vi "ABR-Options Dialog.vi"(0 "Params in":T3={"CAP or ABR"=enum."CAP", "Stimulus"={"Destination"="", "Waveform"=enum."TONE PIP", "Frequency (kHz)"=16.0, "Rep rate (/sec)"=30.0, "Alternate Polarity"=FALSE, "Sampling rate (Hz)"=0.0, "Duration (ms)"=30.0, "Ramp (ms)"=5.0, "Click width (us)"=0.0, "ITI"=enum."Rate", "Save raw"=FALSE}, "Sequence"={"Start (dB)"=20, "Stop (dB)"=80, "Step (dB)"=5}, "Response"={"Gain"=10000, "Averages"=512, "Window (ms)"=8.5, "Thr Fast Steps"=8.5, "Sampling rate (Hz)"=25000.0}} {"Sequence"."Start (dB)" step=5; "Response"."Thr Fast Steps" format="%.2f"; "Response"."Window (ms)" format="%.2f"; "Stimulus"."Frequency (kHz)" format="%.2f"}, 2 "Parent VI":refnum<vi>, 5 "Threshold Estimation In":T2) -> (4 "Params out":T3={"CAP or ABR"=enum."CAP", "Stimulus"={"Destination"="", "Waveform"=enum."TONE PIP", "Frequency (kHz)"=16.0, "Rep rate (/sec)"=30.0, "Alternate Polarity"=FALSE, "Sampling rate (Hz)"=0.0, "Duration (ms)"=30.0, "Ramp (ms)"=5.0, "Click width (us)"=0.0, "ITI"=enum."Rate", "Save raw"=FALSE}, "Sequence"={"Start (dB)"=20, "Stop (dB)"=80, "Step (dB)"=5}, "Response"={"Gain"=10000, "Averages"=512, "Window (ms)"=8.5, "Thr Fast Steps"=8.5, "Sampling rate (Hz)"=25000.0}} {"Sequence"."Start (dB)" step=5; "Response"."Thr Fast Steps" format="%.2f"; "Response"."Window (ms)" format="%.2f"; "Stimulus"."Frequency (kHz)" format="%.2f"}, 6 "Threshold Estimation Out":T2, 8 "Canceled?":bool)   [LabVIEW 2020]
uses:
  Typedefs/ABR-Parameters.ctl
  Typedefs/ABR-Stimulus.ctl
  Typedefs/ABR-Sequence.ctl
  Typedefs/ABR-Response.ctl
  Threshold Estimation VIs/ABR3-Threshold Estimation Parameters.ctl
  epl-vi-lib/Utility VIs/Buttons/KCheckmarkBoolean 2.ctl
panel:
  in  "Save raw data":T1
  out "exit signal":bool
  in  "ITI":enum16{"Rate", "Interval"}(ring) caption="Express intertrial timing as"
  in  "AI Fs":dbl caption="Input sampling rate (Hz)"
  in  "R2 criterion":dbl caption="Adj R2 criterion"
  in  "CC criterion":dbl caption="Corrcoef criterion"
  in  "Thr Tmax":dbl caption="Tmax (ms)"
  in  "Thr Tmin":dbl caption="Tmin (ms)"
  in  "ClickWidth":dbl caption="Click duration (us)"
  in  "ToneRamp":dbl caption="Tone burst ramp length (ms)"
  in  "ToneDur":dbl caption="Tone burst duration (ms)"
  in  "AO Fs":dbl caption="Output sampling rate (Hz)"
  in  "Cancel":bool
  in  "OK":bool
  # "Threshold estimation"
  # "Warning! Unless you're sure you know what you're doing, don't change these parameters"
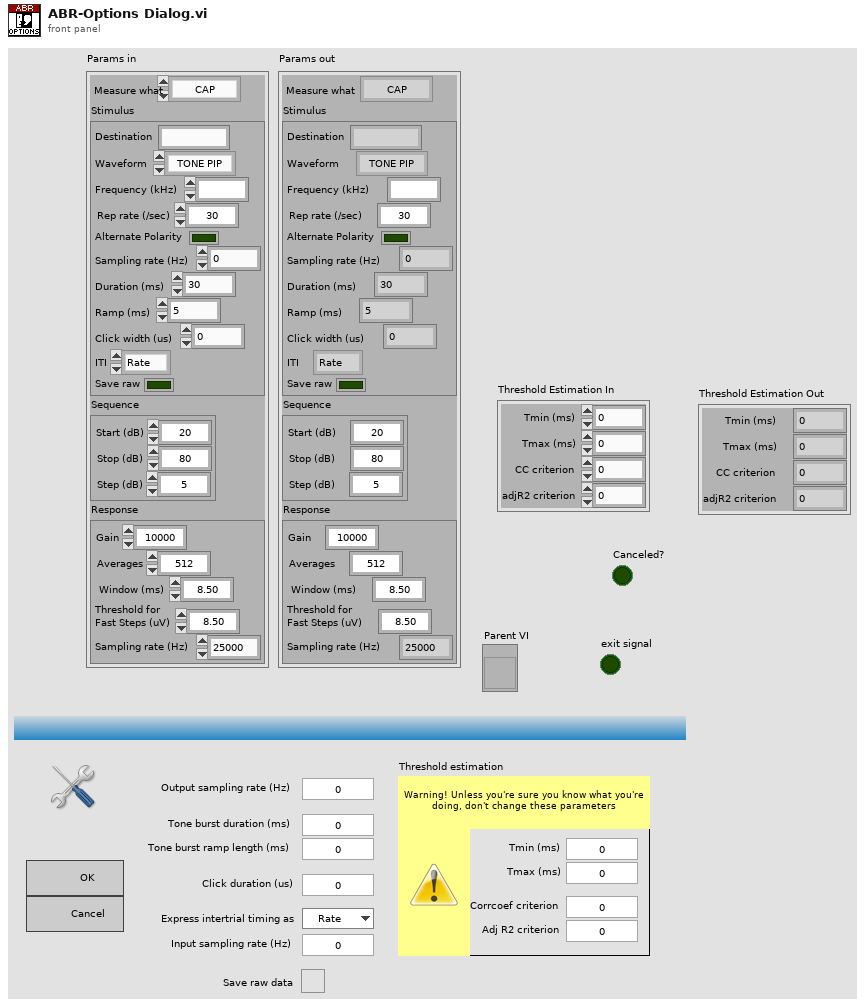
[diagram p1: front panel]
types:
  T1 = typedef "KCheckmarkBoolean 2.ctl" = bool
  T2 = typedef "ABR3-Threshold Estimation Parameters.ctl" = cluster{"Tmin (ms)":dbl, "Tmax (ms)":dbl, "CC criterion":dbl, "adjR2 criterion":dbl}
  T3 = typedef "ABR-Parameters.ctl" = cluster{"CAP or ABR":enum16{"CAP", "ABR"}, "Stimulus":T4, "Sequence":T5, "Response":T6}
  T4 = typedef "ABR-Stimulus.ctl" = cluster{"Destination":string, "Waveform":enum16{"TONE PIP", "CLICK"}, "Frequency (kHz)":ext, "Rep rate (/sec)":dbl, "Alternate Polarity":bool, "Sampling rate (Hz)":dbl, "Duration (ms)":dbl, "Ramp (ms)":dbl, "Click width (us)":dbl, "ITI":enum16{"Rate", "Interval"}, "Save raw":bool}
  T5 = typedef "ABR-Sequence.ctl" = cluster{"Start (dB)":i32, "Stop (dB)":i32, "Step (dB)":i32}
  T6 = typedef "ABR-Response.ctl" = cluster{"Gain":i32, "Averages":i32, "Window (ms)":sgl, "Thr Fast Steps":sgl, "Sampling rate (Hz)":dbl}
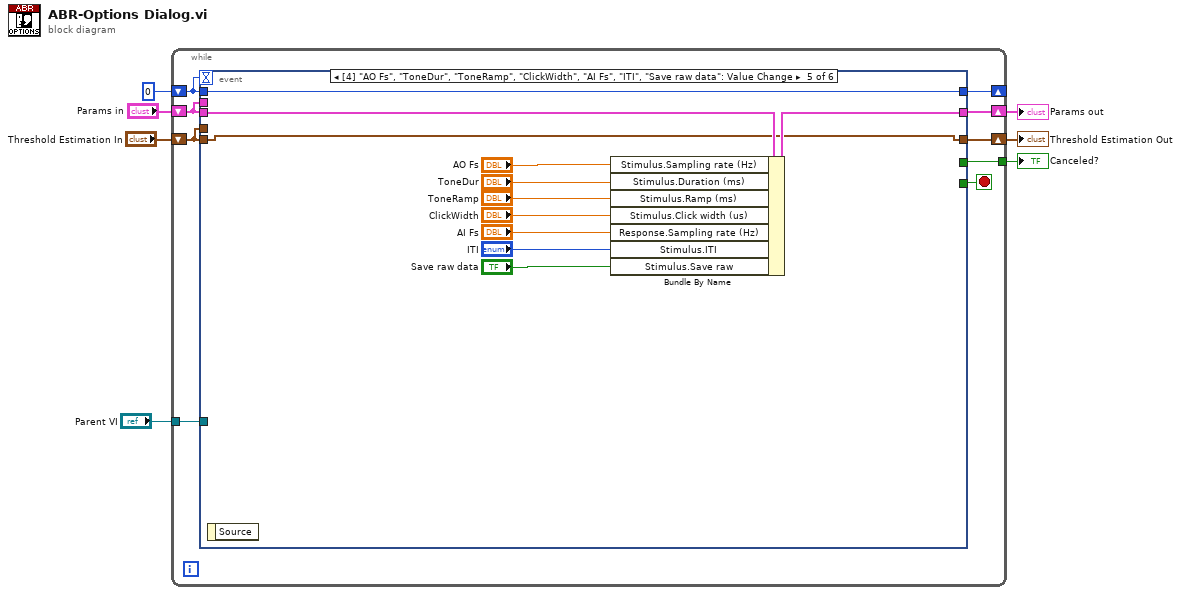
[diagram p0: block diagram]
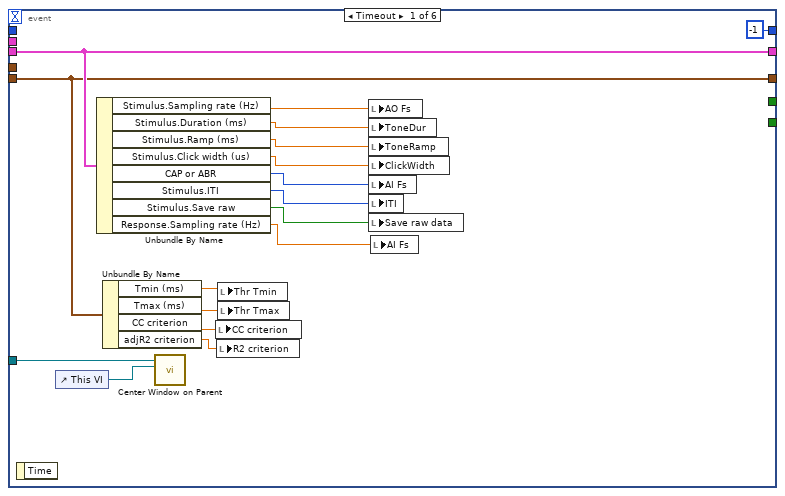
[diagram p2: hidden frame]
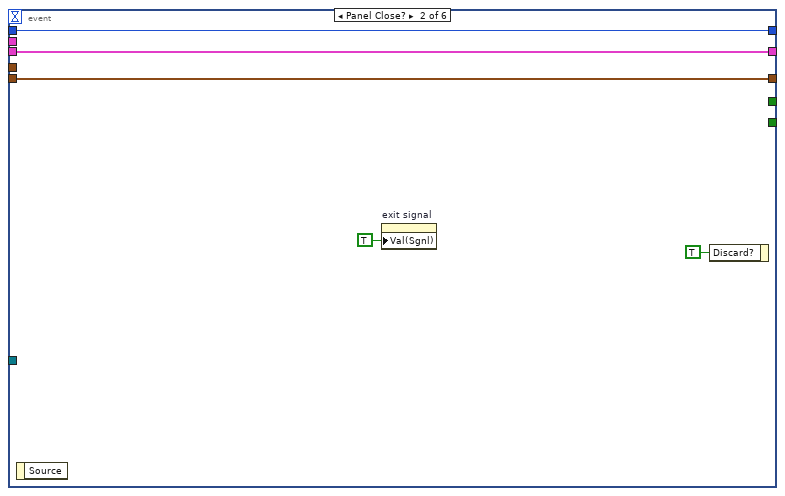
[diagram p3: hidden frame]
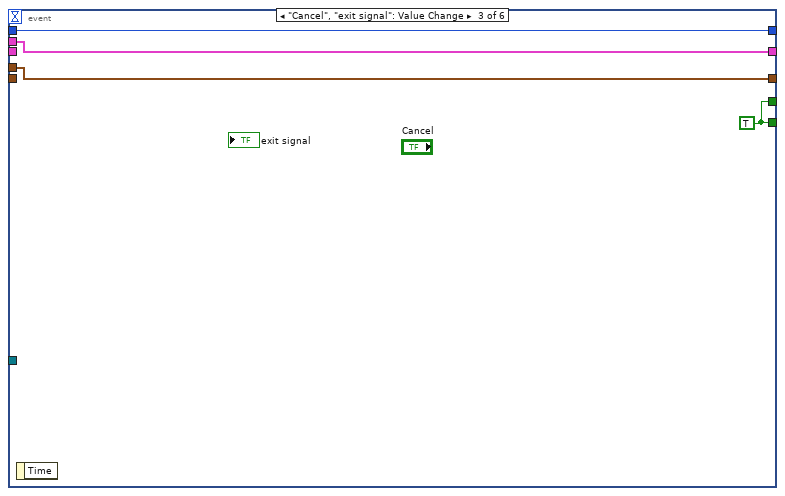
[diagram p4: hidden frame]
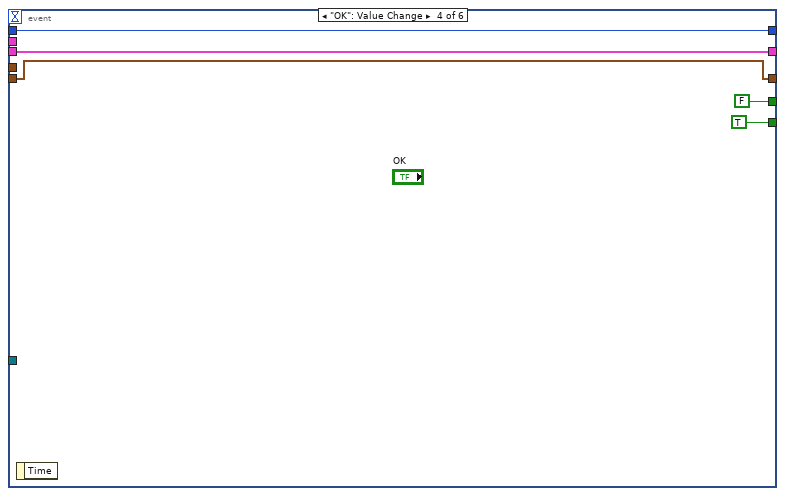
[diagram p5: hidden frame]
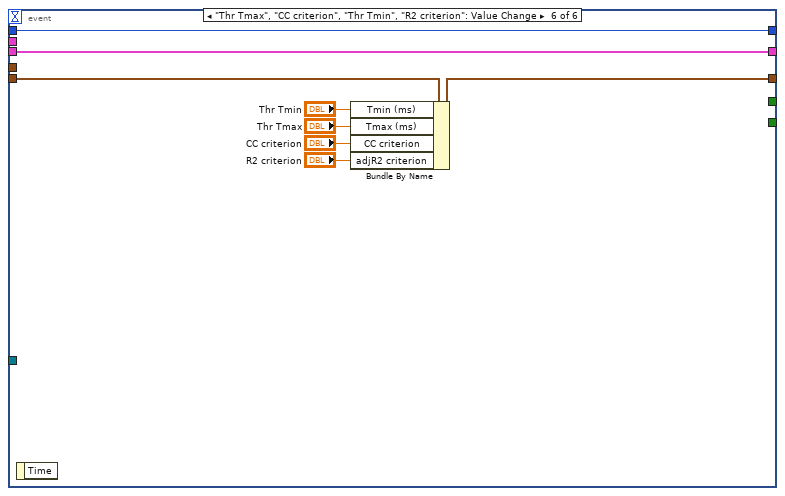
[diagram p6: hidden frame]
diagram:
  n1 = while {
    shift-right: [w16] -> _
    shift-left: 0 -> [w9]
    tunnel: [w13] -> w4
    shift-right: [w15] -> w5
    shift-left: "Params in" -> [w12]
    shift-right: [w11] -> w2
    shift-left: "Threshold Estimation In" -> [w10]
    tunnel: "Parent VI" -> [w8]
    stop <- w14 stop-if-true
    n2 = event shown="[4] \"AO Fs\", \"ToneDur\", \"ToneRamp\", \"ClickWidth\", \"AI Fs\", \"ITI\", \"Save raw data\": Value Change" {
      selector: _ -> [_ _ _ _ _ _]
      dyn-events: _ -> [_ _ _ _ _ _]
      timeout: w9 -> [_ _ _ _ _ _]
      tunnel: [-1 w38 w39 w43 w51 w62] -> w16
      tunnel: w12 -> [w32 w34 _ w47 w58 w66]
      tunnel: [w32 w34 w41 w47 w57 w66] -> w15
      tunnel: [_ _ w42 TRUE _ _] -> w14
      tunnel: [_ _ w42 FALSE _ _] -> w13
      tunnel: w12 -> [_ _ w41 _ _ _]
      tunnel: w10 -> [w27 w37 _ w44 w52 w60]
      tunnel: [w27 w37 w40 w44 w52 w59] -> w11
      tunnel: w10 -> [_ _ w40 _ _ _]
      tunnel: w9 -> [_ w38 w39 w43 w51 w62]
      tunnel: w8 -> [w23 _ _ _ _ _]
      event Timeout {
        n3 = event-data() -> ()  [unwired: 1 in, 1 out]
        n4 = control-ref of="This VI"() -> (w22:refnum<vi>)
        n5 = Unbundle By Name(w32) -> ("Stimulus.Sampling rate (Hz)"=w31:dbl, "Stimulus.Duration (ms)"=w30:dbl, "Stimulus.Ramp (ms)"=w29:dbl, "Stimulus.Click width (us)"=w28:dbl, "CAP or ABR"=w20:enum16{"CAP", "ABR"}, "Stimulus.ITI"=w19:enum16{"Rate", "Interval"}, "Stimulus.Save raw"=w18:bool, "Response.Sampling rate (Hz)"=w17:dbl)
        n6 = Unbundle By Name(w27) -> ("Tmin (ms)"=w26:dbl, "Tmax (ms)"=w25:dbl, "CC criterion"=w24:dbl, "adjR2 criterion"=w21:dbl)
        n7 = call "Center Window on Parent.vi"("Parent VI"=w22, "VI in"=w23) -> ()  [unwired: 8 in, 2 out]
        n8 = local write "CC criterion"(w24) -> ()
        n9 = local write "R2 criterion"(w21) -> ()
        n10 = local write "Thr Tmin"(w26) -> ()
        n11 = local write "Thr Tmax"(w25) -> ()
        n12 = local write "AO Fs"(w31) -> ()
        n13 = local write "ToneDur"(w30) -> ()
        n14 = local write "ToneRamp"(w29) -> ()
        n15 = local write "ClickWidth"(w28) -> ()
        n16 = local write "AI Fs"(w20) -> ()
        n17 = local write "ITI"(w19) -> ()
        n18 = local write "Save raw data"(w18) -> ()
        n19 = local write "AI Fs"(w17) -> ()
      }
      event Panel Close? {
        n20 = event-data() -> ()  [unwired: 1 in, 1 out]
        n21 = property on="exit signal" class="Bool (strict)"("Val(Sgnl)"=TRUE ("Value (Signaling)")) -> ()  [unwired: 2 in, 2 out]
        n22 = event-data("Discard?"=TRUE) -> ()  [unwired: 1 in, 1 out]
      }
      event "Cancel", "exit signal": Value Change {
        w42 = TRUE
        n23 = event-data() -> ()  [unwired: 1 in, 1 out]
      }
      event "OK": Value Change {
        n24 = event-data() -> ()  [unwired: 1 in, 1 out]
      }
      event "AO Fs", "ToneDur", "ToneRamp", "ClickWidth", "AI Fs", "ITI": Value Change {
        n25 = event-data() -> ()  [unwired: 1 in, 1 out]
        n26 = Bundle By Name(cluster=w58, "Stimulus.Sampling rate (Hz)"="AO Fs", "Stimulus.Duration (ms)"="ToneDur", "Stimulus.Ramp (ms)"="ToneRamp", "Stimulus.Click width (us)"="ClickWidth", "Response.Sampling rate (Hz)"="AI Fs", "Stimulus.ITI"="ITI", "Stimulus.Save raw"="Save raw data") -> (w57:T3)
      }
      event "Thr Tmax", "CC criterion", "Thr Tmin", "R2 criterion": Value Change {
        n27 = event-data() -> ()  [unwired: 1 in, 1 out]
        n28 = Bundle By Name(cluster=w60, "Tmin (ms)"="Thr Tmin", "Tmax (ms)"="Thr Tmax", "CC criterion"="CC criterion", "adjR2 criterion"="R2 criterion") -> (w59:T2)
      }
    }
  }
  "Params out" <- w5
  "Canceled?" <- w4
  "Threshold Estimation Out" <- w2
